vi "Display Time Domain and Spectrum.vi"(8 "error in (no error)":errorcluster, 10 "CDB Wfm in":waveform(cdb)) -> (0 "error out":errorcluster, 2 "Power Spectrum / PSD":cluster{"f0":dbl, "df":dbl, "magnitude":dbl[]} {"magnitude" format="%.2p"; "f0" format="%0.2p"; "df" format="%0.2p"}, 3 "I and Q Waveform":waveform(dbl)[](graph) caption="Waveform")   [LabVIEW 2015, in "Monitoring_receiver.lvlib"]
uses:
  Monitoring_receiver.lvlib
  <vilib>/Analysis/4window.llb/windowTd.ctl
  <vilib>/measure/maspectr.llb/FFT Power Spectrum and PSD for 1 Chan (CDB).vi
  <vilib>/measure/NI_MAPro.lvlib
  <vilib>/Analysis/NI_AALPro.lvlib
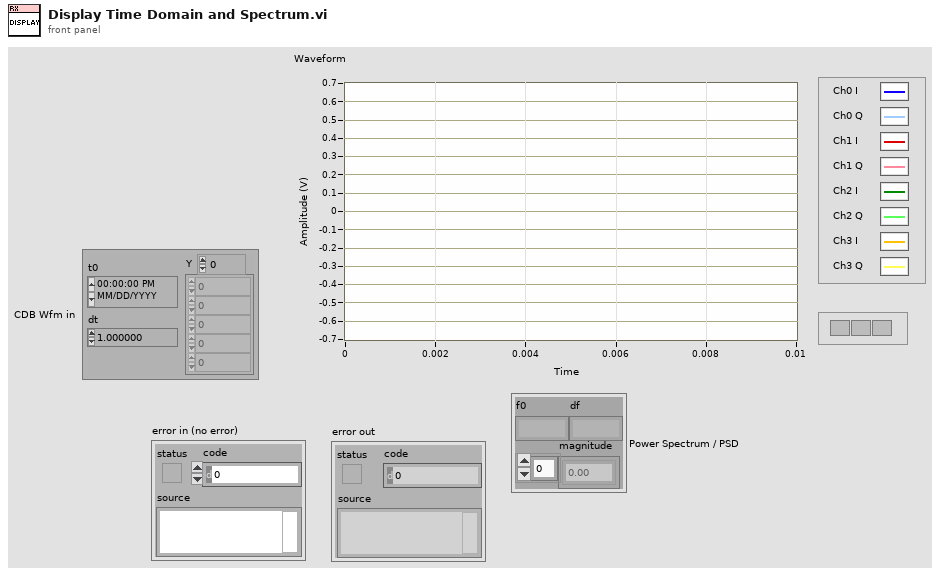
[diagram p1: front panel]
types:
  T1 = cluster{"averaging mode":enum16{"No averaging", "Vector averaging", "RMS averaging", "Peak hold"}, "weighting mode":enum16{"Linear", "Exponential"}, "number of averages":u32}
  T2 = typedef "NI_AALPro.lvlib/windowTd.ctl" = u32
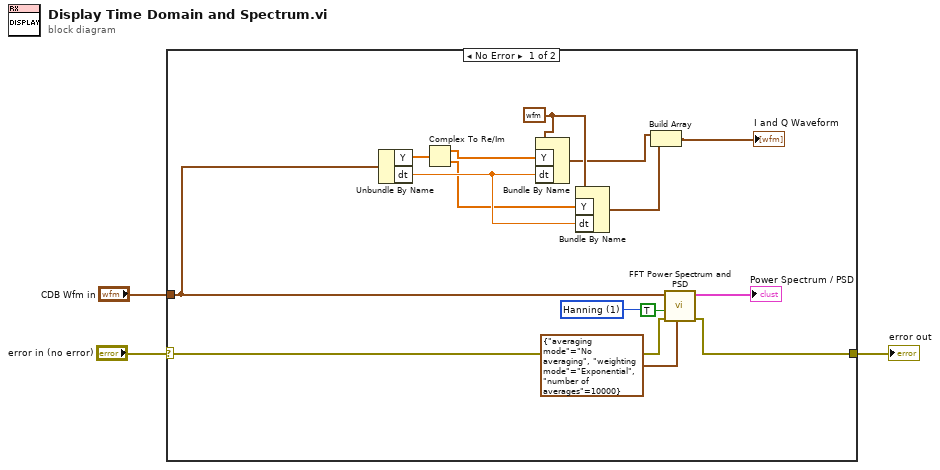
[diagram p0: block diagram]
diagram:
  n1 = case shown="No Error" "error in (no error)" {
    selector: "error in (no error)" -> [w7 w19]
    tunnel: [w17 w19] -> w3
    tunnel: "CDB Wfm in" -> [w13 _]
    frame No Error {
      w8 = waveform(dbl) {"t0"=timestamp(0 s since 1904-01-01), "dt"=1.0, "Y"=[]} ("new element/subarray")
      w15 = T2 1 items=["Rectangle"=0, "Hanning"=1, "Hamming"=2, "Blackman-Harris"=3, "Exact Blackman"=4, "Blackman"=5, "Flat Top"=6, "4 Term B-Harris "=7, "7 Term B-Harris"=8, "Low Sidelobe"=9, "Blackman Nuttall"=11, "Triangle"=30, "Bartlett-Hanning"=31, "Bohman"=32, "Parzen"=33, "Welch"=34, "Kaiser"=60, "Dolph-Chebyshev"=61, "Gaussian"=62] ("window")
      n2 = Unbundle By Name(w13) -> ("Y"=w11:cdb[], "dt"=w12:dbl)
      n3 = Complex To Re/Im(x + iy=w11) -> (x=w10:dbl[], y=w9:dbl[])
      n4 = Bundle By Name(cluster=w8, "Y"=w10, "dt"=w12) -> (w6:waveform(dbl))
      n5 = Bundle By Name(cluster=w8, "Y"=w9, "dt"=w12) -> (w5:waveform(dbl))
      n6 = Build Array(w6, w5) -> (→"I and Q Waveform":waveform(dbl)[])
      n7 = call-poly <vilib>:"FFT Power Spectrum and PSD.vi"("averaging parameters"=T1 {"averaging mode"=enum."No averaging", "weighting mode"=enum."Exponential", "number of averages"=10000}, "error in (no error)"=w7, "dB On (F)"=TRUE, "window"=w15, "time signal"=w13) -> ("error out"=w17:errorcluster, "Power Spectrum / PSD"=→"Power Spectrum / PSD":cluster{"f0":dbl, "df":dbl, "magnitude":dbl[]})  [unwired: 3 in, 2 out]
    }
    frame Error {
    }
  }
  "error out" <- w3
